vi "CheckStartEndCount.vi"(8 "End channel":string="116", 11 "Start channel":string="101") -> (1 "Length string":string, 2 "Length number":i32)   [LabVIEW 2013]
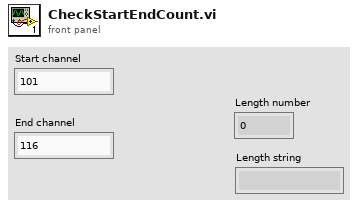
[diagram p1: front panel]
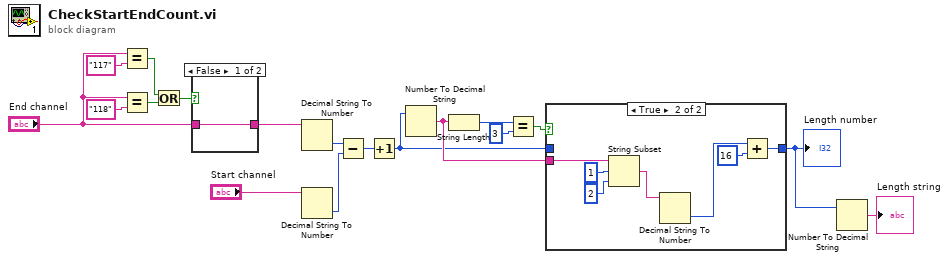
[diagram p0: block diagram]
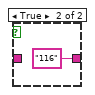
[diagram p2: hidden frame]
diagram:
  n1 = Equal?(x="End channel", y="117") -> (x = y?=w7:bool)
  n2 = Equal?(x="End channel", y="118") -> (x = y?=w8:bool)
  n3 = Or(x=w7, y=w8) -> (x .or. y?=w6:bool)
  n4 = case shown="False" w6 {
    tunnel: [w19 "116"] -> w4
    tunnel: "End channel" -> [w19 _]
    frame False {
    }
    frame True {
    }
  }
  n5 = Decimal String To Number(string=w4) -> (number=w18:i32)  [unwired: 2 in, 1 out]
  n6 = Decimal String To Number(string="Start channel") -> (number=w17:i32)  [unwired: 2 in, 1 out]
  n7 = Subtract(x=w18, y=w17) -> (x-y=w16:i32)
  n8 = Increment(x=w16) -> (x+1=w11:i32)
  n9 = Number To Decimal String(number=w11) -> (decimal integer string=w12:string)  [unwired: 1 in]
  n10 = String Length(string=w12) -> (length=w15:i32)
  n11 = Equal?(x=w15, y=3) -> (x = y?=w13:bool)
  n12 = case shown="True" w13 {
    tunnel: w12 -> [_ w28]
    tunnel: [w21 w22] -> w2
    tunnel: w11 -> [w21 _]
    frame False {
    }
    frame True {
      n13 = String Subset(string=w28, offset (0)=1, length (rest)=2 ("length (rest)")) -> (substring=w25:string)
      n14 = Decimal String To Number(string=w25) -> (number=w24:i32)  [unwired: 2 in, 1 out]
      n15 = Add(x=w24, y=16) -> (x+y=w22:i32)
    }
  }
  "Length number" <- w2
  n16 = Number To Decimal String(number=w2) -> (decimal integer string=→"Length string":string)  [unwired: 1 in]
